vi "Teleop.vi"(10 "Match Info":T1={"Autonomous Elapsed Seconds"=0.0, "TeleOp Elapsed Seconds"=0.0, "Disabled Elapsed Seconds"=0.0, "Visited Autonomous"=FALSE, "Visited TeleOp"=FALSE, "Visited Disabled"=FALSE, "Autonomous Settings"={"Autonomous Style"=enum."Independent", "VI Refnum"=refnum}}, 11 "Call Context":T2) -> ()   [LabVIEW 2015]
doc: "This VI is called for each TeleOp packet received from the DS where the robot is not disabled. It is often used to read from the joysticks and update I/O or to update setpoints for timed control loops. It should complete and return within 20 milliseconds or it may miss DS packets."
uses:
  <vilib>/Rock Robotics/WPI/DriverStation/WPI_DriverStationDerivedRobotMode.ctl
  <vilib>/Rock Robotics/WPI/DriverStation/WPI_DriverStationMatch Info.ctl
  <vilib>/Rock Robotics/WPI/RobotDrive/WPI_RobotDriveGetSetRefNum.vi
  <vilib>/Rock Robotics/WPI/Joystick/WPI_JoystickGetSetRefNum.vi
  Robot Global Data.vi
panel:
  in  "Quickturn_Sens_Low":dbl=1.0
  in  "QuickTurn Const":dbl=0.25
  in  "Speedturn_Sens_Low":dbl=0.75
  out "Sample Slider 0":dbl(slide) scale=0.0..5.0
  out "Sample Boolean 1":bool
  out "Sample Boolean 0":bool
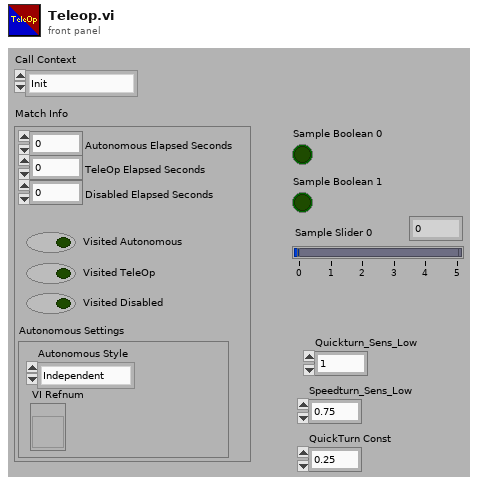
[diagram p1: front panel]
types:
  T1 = typedef "WPI_DriverStationMatch Info.ctl" = cluster{"Autonomous Elapsed Seconds":dbl, "TeleOp Elapsed Seconds":dbl, "Disabled Elapsed Seconds":dbl, "Visited Autonomous":bool, "Visited TeleOp":bool, "Visited Disabled":bool, "Autonomous Settings":cluster{"Autonomous Style":enum16{"Iterative", "Independent"}, "VI Refnum":refnum<vi>}}
  T2 = typedef "WPI_DriverStationDerivedRobotMode.ctl" = enum16{"Init", "Execute", "Stop"}
  T3 = typedef "WPI_JoystickDevRef.ctl" = cluster{"Device":T4}
  T4 = typedef "WPI_JoystickDeviceEnum.ctl" = enum16{"USB 0", "USB 1", "USB 2", "USB 3", "USB 4", "USB 5"}
  T5 = typedef "WPI_RobotDriveDevRef.ctl" = cluster{"DevStatus":errorcluster, "Motors[]":T6[], "Square Inputs":bool, "Max Output":dbl}
  T6 = typedef "WPI_MotorControlDeviceRef.ctl" = cluster{"DeviceStatus":errorcluster, "Type":enum16{"PWM", "CAN"}, "PWM":cluster{"Digital Module":T7, "PWM Channel":T8, "DeadBand":T9}, "CAN":cluster{"Device Number":u8, "Control Mode":T10, "Semaphore":T11, "Max Vout":dbl}, "Invert":bool, "TransformRef":T12, "InvTransformRef":T12}
  T7 = typedef "FPGA_TypedefDigitalModule.ctl" = enum16{"Digital Module 1", "Digital Module 2"}
  T8 = typedef "FPGA_DIOPWMChannel.ctl" = enum8{"PWM 1", "PWM 2", "PWM 3", "PWM 4", "PWM 5", "PWM 6", "PWM 7", "PWM 8", "PWM 9", "PWM 10", "Invalid"}
  T9 = typedef "WPI_PWMDeadband.ctl" = cluster{"Name":string, "maxPositivePwm":i32, "minPositivePwm":i32, "centerPwm":i32, "maxNegativePwm":i32, "minNegativePwm":i32, "angularRange":u16}
  T10 = typedef "WPI_CANJaguar_ControlMode.ctl" = enum8{"Percent VBus", "Current", "Speed", "Position", "Voltage"}
  T11 = typedef "Semaphore RefNum" = refnum<k1>
  T12 = typedef "WPI_PWMTransform_ConPane.ctl" = refnum<vi>
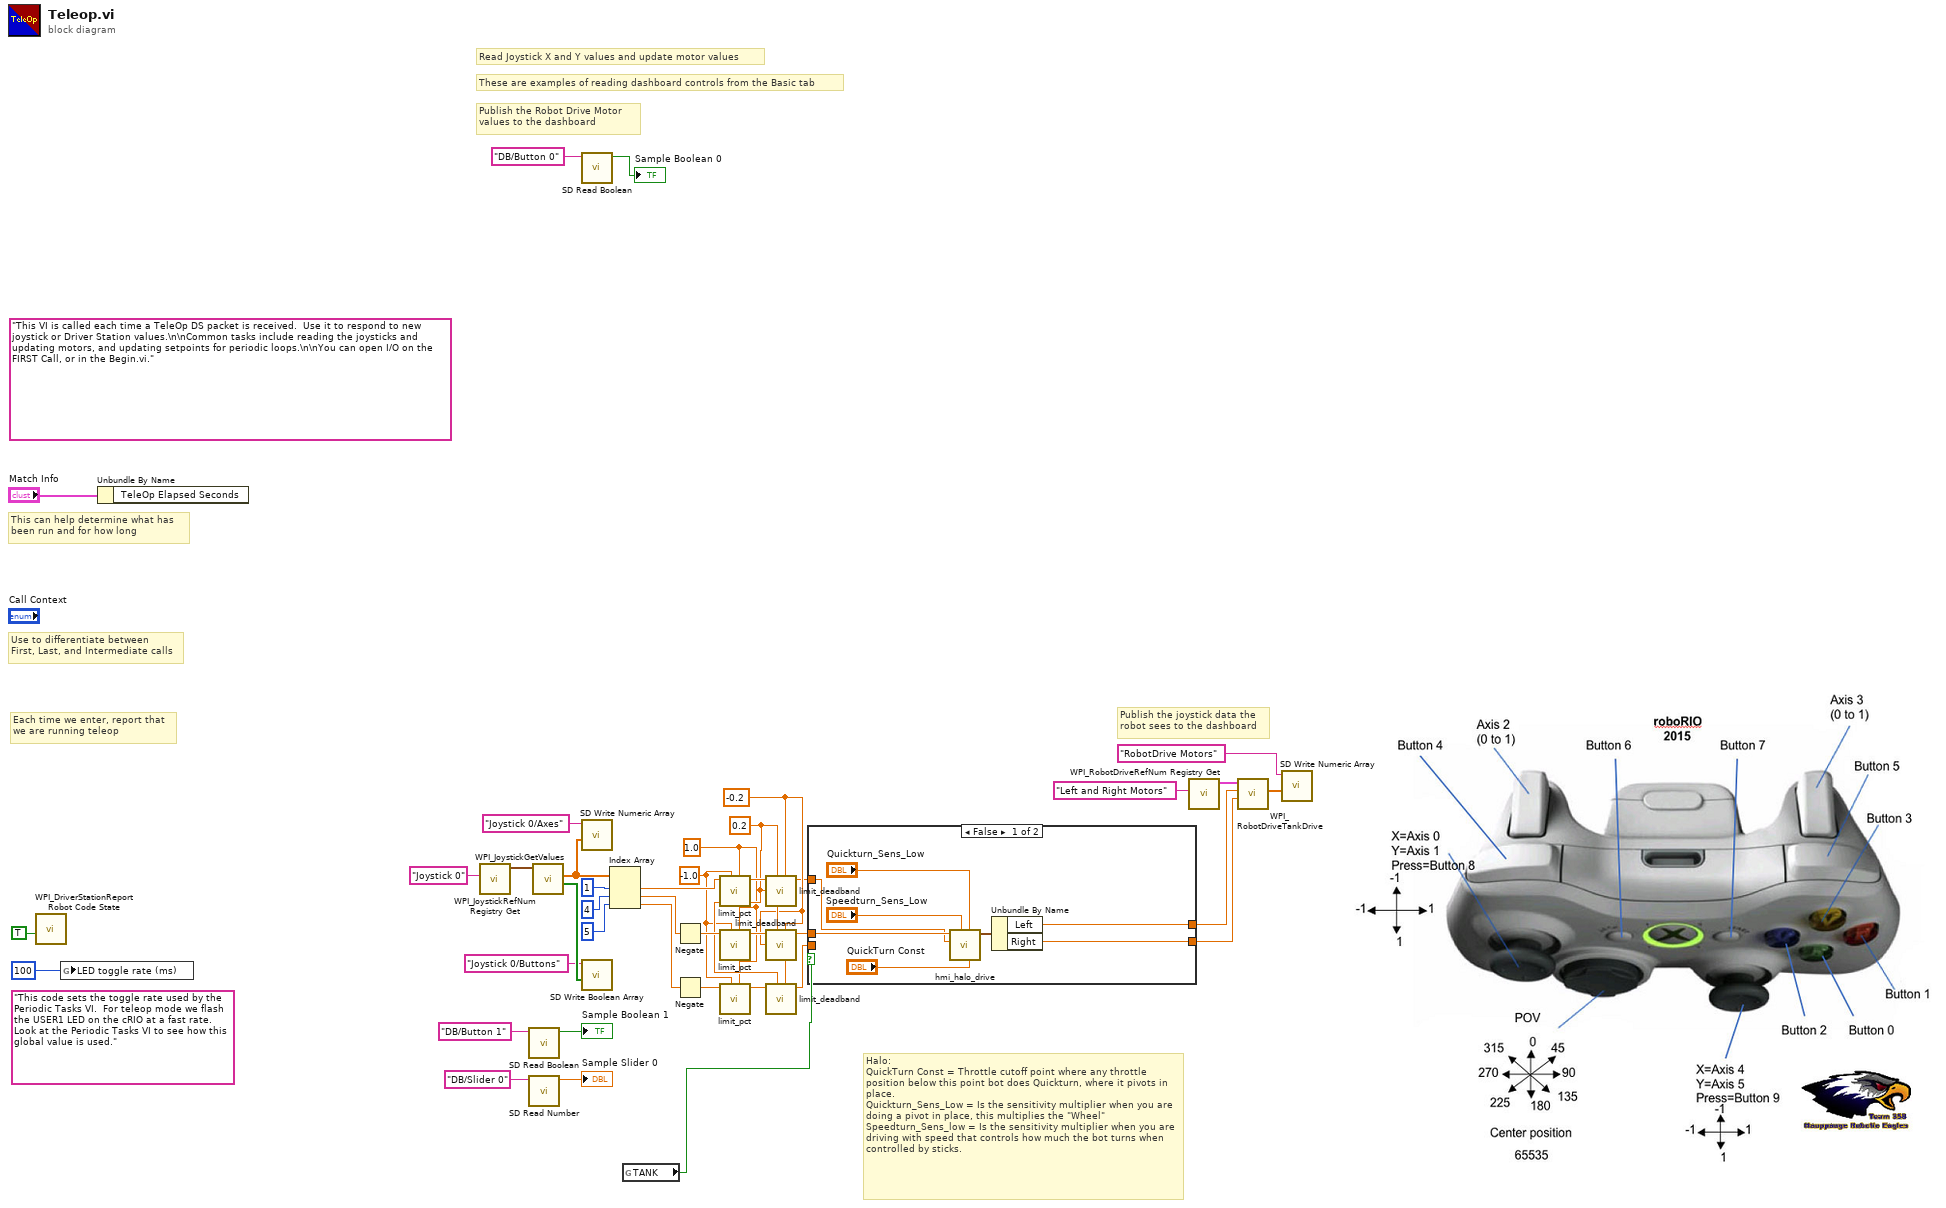
[diagram p0: block diagram]
diagram:
  w10 = 1.0 ("upper limit")
  w2 = -1.0 ("lower limit")
  w11 = -0.2 ("lower limit")
  w12 = 0.2 ("upper limit")
  (unwired) "This code sets the toggle rate used by the Periodic Tasks VI.  For teleop mode we flash the USER1 LED on the cRIO at a fast rate.  Look at the Periodic Tasks VI to see how this global value is used."
  (unwired) "This VI is called each time a TeleOp DS packet is received.  Use it to respond to new joystick or Driver Station values.\n\nCommon tasks include reading the joysticks and updating motors, and updating setpoints for periodic loops.\n\nYou can open I/O on the FIRST Call, or in the Begin.vi."
  # "Halo:\nQuickTurn Const = Throttle cutoff point where any throttle position below this point bot does Quickturn, where it pivots in place.\nQuickturn_Sens_Low = Is the sensitivity multiplier when you are doing a pivot in place, this multiplies the \"Wheel\" \nSpeedturn_Sens_low = Is the sensitivity multiplier when you are driving with speed that controls how much the bot turns when controlled by sticks."
  # "These are examples of reading dashboard controls from the Basic tab"
  # "Publish the Robot Drive Motor\nvalues to the dashboard"
  # "Publish the joystick data the\nrobot sees to the dashboard"
  # "Each time we enter, report that\nwe are running teleop"
  # "Use to differentiate between\nFirst, Last, and Intermediate calls"
  # "This can help determine what has\nbeen run and for how long"
  # "Read Joystick X and Y values and update motor values"
  n1 = call <vilib>:"WPI_DriverStationReport Robot Code State.vi"("TeleOp"=TRUE ("Autonomous")) -> ()  [unwired: 10 in, 1 out]
  n2 = global write "Robot Global Data.vi" "LED toggle rate (ms)"(u32 100 ("LED ms toggle rate")) -> ()
  n3 = Unbundle By Name("Match Info") -> ()  [unwired: 1 out]
  n4 = call <vilib>:"WPI_JoystickRefNum Registry Get.vi"("refnum name"="Joystick 0") -> ("JoystickDevRef"=w37:T3)  [unwired: 1 in, 9 out]
  n5 = call <vilib>:"SD Read Boolean.vi"("Name"="DB/Button 1" ("refnum name")) -> ("Boolean"=→"Sample Boolean 1":bool)  [unwired: 8 in, 2 out]
  n6 = call <vilib>:"SD Read Number.vi"("Name"="DB/Slider 0" ("refnum name")) -> ("Numeric"=→"Sample Slider 0":dbl)  [unwired: 8 in, 2 out]
  n7 = call <vilib>:"WPI_JoystickGetValues.vi"("JoystickDevRef"=w37) -> ("Buttons"=w34:bool[], "Axes"=w24:dbl[])  [unwired: 6 in, 3 out]
  n8 = call <vilib>:"SD Read Boolean.vi"("Name"="DB/Button 0" ("refnum name")) -> ("Boolean"=→"Sample Boolean 0":bool)  [unwired: 8 in, 2 out]
  n9 = call <vilib>:"SD Write Numeric Array.vi"("Numeric Array"=w24, "Name"="Joystick 0/Axes") -> ()  [unwired: 8 in, 2 out]
  n10 = call <vilib>:"SD Write Boolean Array.vi"("Boolean Array"=w34, "Name"="Joystick 0/Buttons") -> ()  [unwired: 8 in, 2 out]
  n11 = Index Array(array=w24, index #1=1 ("index"), index #2=4 ("index"), index #3=5 ("index")) -> (element #1=w19:dbl, element #2=w15:dbl, element #3=w5:dbl)
  n12 = global read "Robot Global Data.vi" "TANK"() -> (w1:bool)
  n13 = Negate(x=w15) -> (-x=w14:dbl)
  n14 = Negate(x=w5) -> (-x=w4:dbl)
  n15 = call "limit_pct.vi"("upper limit"=w10, "lower limit"=w2, "PCT"=w19) -> ("PCT Out"=w22:dbl)  [unwired: 8 in]
  n16 = call "limit_pct.vi"("upper limit"=w10, "lower limit"=w2, "PCT"=w14) -> ("PCT Out"=w23:dbl)  [unwired: 8 in]
  n17 = call "limit_pct.vi"("upper limit"=w10, "lower limit"=w2, "PCT"=w4) -> ("PCT Out"=w13:dbl)  [unwired: 8 in]
  n18 = call "limit_deadband.vi"("lower limit"=w11, "upper limit"=w12, "Val"=w22) -> ("Val Out"=w7:dbl)  [unwired: 8 in]
  n19 = call "limit_deadband.vi"("lower limit"=w11, "upper limit"=w12, "Val"=w23) -> ("Val Out"=w8:dbl)  [unwired: 8 in]
  n20 = call "limit_deadband.vi"("lower limit"=w11, "upper limit"=w12, "Val"=w13) -> ("Val Out"=w3:dbl)  [unwired: 8 in]
  n21 = case shown="False" w1 {
    tunnel: [w47 w49] -> w9
    tunnel: w8 -> [w46 w50]
    tunnel: w7 -> [w45 _]
    tunnel: [w44 w50] -> w6
    tunnel: w3 -> [_ w49]
    frame False {
      n22 = call "hmi_halo_drive.vi"("QuickTurn Const"="QuickTurn Const", "Quickturn_Sens_Low"="Quickturn_Sens_Low", "Speedturn_Sens_Low"="Speedturn_Sens_Low", "Wheel"=w45, "Throttle"=w46) -> ("Drive Data"=w48:cluster{"Left":dbl, "Right":dbl})  [unwired: 6 in]
      n23 = Unbundle By Name(w48) -> ("Left"=w44:dbl, "Right"=w47:dbl)
    }
    frame True {
    }
  }
  n24 = call <vilib>:"WPI_RobotDriveRefNum Registry Get.vi"("refnum name"="Left and Right Motors") -> ("RobotDriveDevRef"=w20:T5)  [unwired: 1 in, 9 out]
  n25 = call <vilib>:"WPI_RobotDriveTankDrive.vi"("Right axis value"=w9, "Left axis value"=w6, "RobotDriveDevRef"=w20) -> ("Motor Values"=w21:dbl[])  [unwired: 6 in, 2 out]
  n26 = call <vilib>:"SD Write Numeric Array.vi"("Numeric Array"=w21, "Name"="RobotDrive Motors") -> ()  [unwired: 8 in, 2 out]
